vi "Receive Shortcut Menu Selection Event.vi"(8 "error in (no error)":errorcluster, 10 "ShortcutMenuSelectionMsg":refnum<class "ShortcutMenuSelectionMsg.lvclass">, 11 "TreeActor In":refnum<class "TreeActor.lvclass">) -> (0 "error out":errorcluster, 3 "TreeActor Out":refnum<class "TreeActor.lvclass">)   [LabVIEW 2017, in "TestViewables.lvlib" / "TreeActor.lvclass"]
doc: "<License>\nCopyright © 2017 Composed Systems, LLC | All rights reserved\nwww.composed.io\n\nAuthor: Ethan Stern <ethan.stern@composed.io>\n\nThis software is provided \"AS IS\" WITHOUT WARRANTIES, either express or implied, AND IS FOR EDUCATIONAL PURPOSES ONLY.\n</License>"
uses:
  TreeActor.lvclass
  C:/Git/mva-framework/Source/Framework/IViewable/IViewable/IViewable.lvclass
  Source/Framework/ActorEvents/IEventAggregator Messages/ShortcutMenuSelectionMsg/ShortcutMenuSelectionMsg.lvclass
  Source/Framework/ActorEvents/IEventAggregator Messages/ShortcutMenuSelectionMsg/ShortcutMenuSelectionMsg.lvclass/ShortcutMenuSelectionMsg.ctl
  Source/Framework/ActorEvents/IEventAggregator Messages/ShortcutMenuSelectionMsg/Accessors/Read Item Tag.vi
  Source/DialogBox/OneButtonDialogBox/OneButtonDialogBox.lvclass
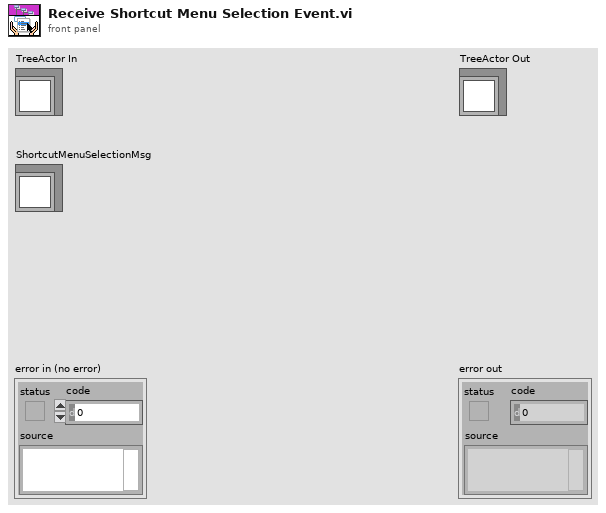
[diagram p1: front panel]
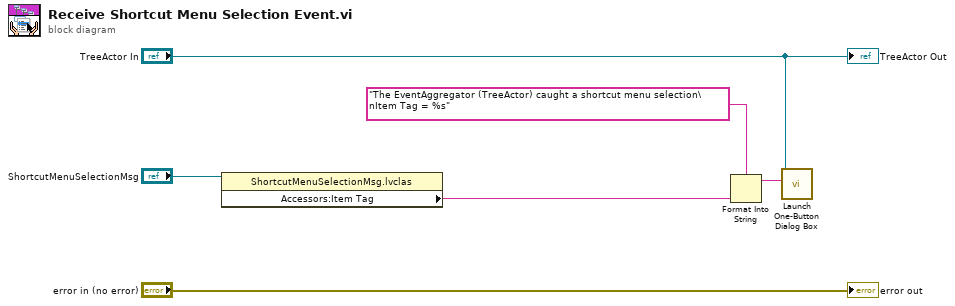
[diagram p0: block diagram]
diagram:
  n1 = property class="ShortcutMenuSelectionMsg.lvclas"(reference="ShortcutMenuSelectionMsg") -> ("Accessors:Item Tag"=w1:string)  [unwired: 1 in, 2 out]
  n2 = Format Into String(format string="The EventAggregator (TreeActor) caught a shortcut menu selection\nItem Tag = %s", w1) -> (resulting string=w2:string)  [unwired: 2 in, 1 out]
  n3 = call "Launch One-Button Dialog Box.vi"("Message Text"=w2, "Dialog Launcher"="TreeActor In") -> ()  [unwired: 9 in, 1 out]
  "error out" <- "error in (no error)"
  "TreeActor Out" <- "TreeActor In"
